vi "CollectorWrap.vi"(7 "Action":T1=enum."Collect", 8 "error in":errorcluster) -> (0 "error out":errorcluster)   [LabVIEW 2015]
doc: "Wrapper for collecting. It has the following actions:\n-Stop: turns the roller motor off. Raises the arm for a small amount of time, then stops the arm.\n-PreCollect: actuates the clapper to middle, the roller pneumatic to middle, and spins the roller motor forward.\n-Collect: actuates the clapper to in."
uses:
  CollectorWrapAction.ctl
  DoubleSolenoidAction.ctl
  RollerAction.ctl
  CollectorAction.ctl
panel:
  in  "RaiseArmSpeed":dbl=1.0
  in  "RaiseArmWait":u32=200
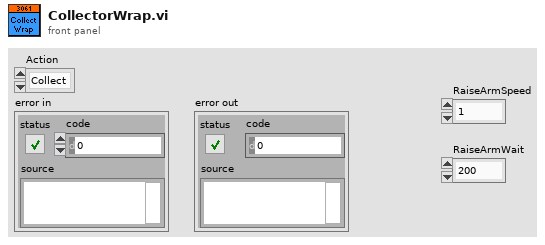
[diagram p1: front panel]
types:
  T1 = typedef "CollectorWrapAction.ctl" = enum16{"Stop", "PreCollect", "Collect"}
  T2 = typedef "DoubleSolenoidAction.ctl" = enum16{"Init", "Middle", "In", "Out"}
  T3 = typedef "CollectorAction.ctl" = enum16{"Init", "Raise", "Lower", "Stop", "GetStatus"}
  T4 = typedef "RollerAction.ctl" = enum16{"Init", "Off", "Forward", "Reverse"}
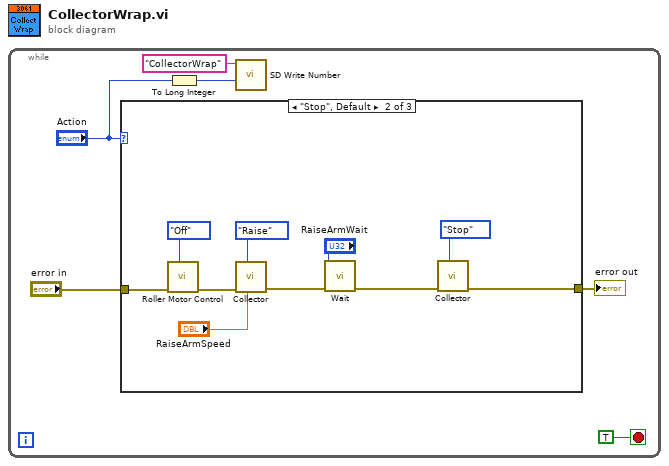
[diagram p0: block diagram]
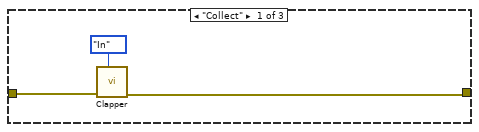
[diagram p2: hidden frame]
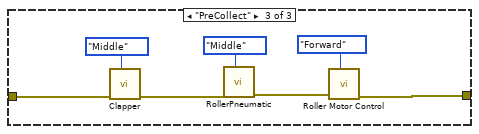
[diagram p3: hidden frame]
diagram:
  n1 = while {
    stop <- TRUE stop-if-true
    n2 = case shown="\"Stop\", Default" "Action" {
      tunnel: "error in" -> [w9 w19 w24]
      tunnel: [w8 w11 w26] -> w4
      frame "Collect" {
        n3 = call "Clapper.vi"("State"=DoubleSolenoidAction."In", "Error in"=w9) -> ("Error out"=w8:errorcluster)  [unwired: 9 in]
      }
      frame "Stop", Default {
        n4 = call "Roller Motor Control.vi"("Action"=RollerAction."Off", "Error in"=w19) -> ("Error out"=w17:errorcluster)  [unwired: 9 in]
        n5 = call "Collector.vi"("MotorSpeed"="RaiseArmSpeed", "Action"=CollectorAction."Raise", "Error in"=w17) -> ("Error out"=w15:errorcluster)  [unwired: 6 in, 2 out]
        n6 = call "Wait.vi"("error in"=w15, "milliseconds to wait"="RaiseArmWait") -> ("error out"=w12:errorcluster)  [unwired: 9 in]
        n7 = call "Collector.vi"("Action"=CollectorAction."Stop", "Error in"=w12) -> ("Error out"=w11:errorcluster)  [unwired: 7 in, 2 out]
      }
      frame "PreCollect" {
        n8 = call "Clapper.vi"("State"=DoubleSolenoidAction."Middle", "Error in"=w24) -> ("Error out"=w23:errorcluster)  [unwired: 9 in]
        n9 = call "RollerPneumatic.vi"("State"=DoubleSolenoidAction."Middle", "Error in"=w23) -> ("Error out"=w22:errorcluster)  [unwired: 9 in]
        n10 = call "Roller Motor Control.vi"("Action"=RollerAction."Forward", "Error in"=w22) -> ("Error out"=w26:errorcluster)  [unwired: 9 in]
      }
    }
    "error out" <- w4
    n11 = To Long Integer(number="Action") -> (32bit integer=w3:i32)
    n12 = call <vilib>:"SD Write Number.vi"("Numeric"=w3, "Name"="CollectorWrap") -> ()  [unwired: 8 in, 2 out]
  }
